vi "EnableDisable.vi"() -> ()   [LabVIEW 2011, in "IVI DC Power Supply Custom Device.lvlib"]
uses:
  IVI DC Power Supply Custom Device.lvlib
  <vilib>/NI Veristand/Custom Device API/Custom Device Item Ref.ctl
  <vilib>/NI Veristand/Custom Device API/Custom Device API.lvlib
panel:
  in  "Node Ptr":T1=18446744073709551615 format="%.0x"
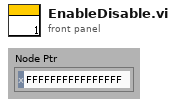
[diagram p1: front panel]
types:
  T1 = typedef "Custom Device API.lvlib/Custom Device Item Ref.ctl" = u64
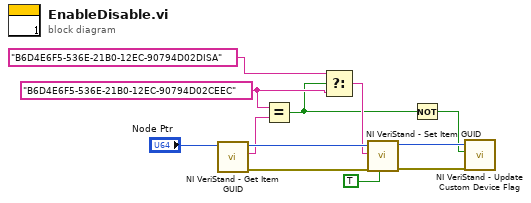
[diagram p0: block diagram]
diagram:
  w5 = "B6D4E6F5-536E-21B0-12EC-90794D02CEEC"
  n1 = call <vilib>:"NI VeriStand - Get Item GUID.vi"("Item Ref in"="Node Ptr") -> ("error out"=w11:errorcluster, "GUID"=w6:string, "Item Ref out"=w9:T1)  [unwired: 8 in]
  n2 = Equal?(x=w5, y=w6) -> (x = y?=w2:bool)
  n3 = Select(t="B6D4E6F5-536E-21B0-12EC-90794D02DISA", s=w2, f=w5) -> (s? t:f=w3:string)
  n4 = call <vilib>:"NI VeriStand - Set Item GUID.vi"("Refresh System Explorer Tree? (F)"=TRUE, "error in (no error)"=w11, "GUID"=w3, "Item Ref in"=w9) -> ("error out"=w8:errorcluster, "Item Ref out"=w7:T1)  [unwired: 6 in]
  n5 = Not(x=w2) -> (.not. x?=w1:bool)
  n6 = call <vilib>:"NI VeriStand - Update Custom Device Flag.vi"("error in (no error)"=w8, "Is Custom Device Active?"=w1, "Device Ref in"=w7) -> ()  [unwired: 7 in, 2 out]
